vi "Add Reply Messenger.vi"(8 "error in (no error)":errorcluster, 10 "Reply to...":refnum<class "Send.lvclass">, 11 "Message":refnum<class "MSG.lvclass">) -> (0 "error out":errorcluster, 2 "Reply to...":refnum<class "Send.lvclass">, 3 "Message":refnum<class "MSG.lvclass">)   [LabVIEW 2011, in "Messenging.lvlib" / "MSG.lvclass"]
uses:
  MSG.lvclass
  Send/Send.lvclass
  MSG.lvclass/MSG.ctl
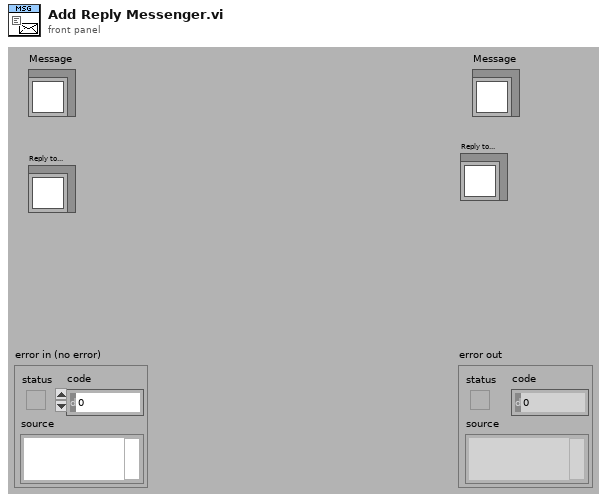
[diagram p1: front panel]
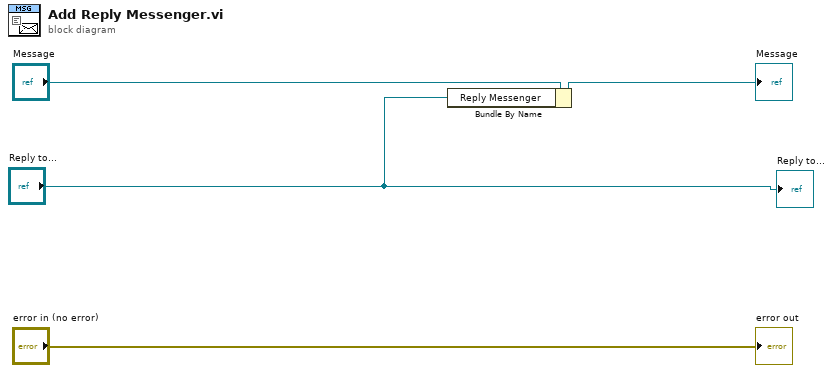
[diagram p0: block diagram]
diagram:
  n1 = Bundle By Name(cluster="Message", "Reply Messenger"="Reply to...") -> (→"Message":refnum<class "MSG.lvclass">)
  "error out" <- "error in (no error)"
  "Reply to..." <- "Reply to..."
